vi "set_z_voltage.vi"(8 "error in (no error)":errorcluster, 10 "Z voltage (bits)":i16, 11 "PZT in":refnum<class "PZT.lvclass">) -> (0 "error out":errorcluster, 3 "PZT out":refnum<class "PZT.lvclass">)   [LabVIEW 2020, in "PZT.lvclass"]
uses:
  PZT.lvclass
  PZT.lvclass/PZT.ctl
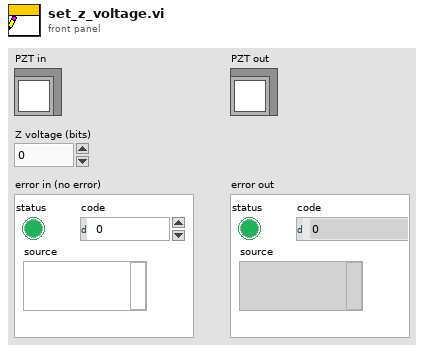
[diagram p1: front panel]
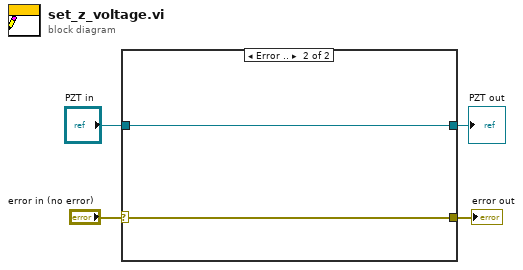
[diagram p0: block diagram]
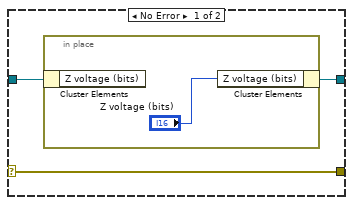
[diagram p2: hidden frame]
diagram:
  n1 = case shown="Error .." "error in (no error)" {
    selector: "error in (no error)" -> [w5 w10]
    tunnel: "PZT in" -> [w7 w9]
    tunnel: [w6 w9] -> w3
    tunnel: [w5 w10] -> w1
    frame No Error {
      n2 = in-place {
        n3 = in-place-cluster #1(w7) -> ()  [unwired: 1 out]
        n4 = in-place-cluster #1("Z voltage (bits)"="Z voltage (bits)") -> (w6:refnum<class "PZT.lvclass">)
      }
    }
    frame Error {
    }
  }
  "error out" <- w1
  "PZT out" <- w3
